vi "DestroyClone.vi"(8 "error in (no error)":errorcluster, 9 "Exit via Stop Module Req?":bool, 10 "Wait for Module to stop?":bool, 11 "ModuleAdmin":refnum<class "ModuleAdmin.lvclass">) -> (0 "error out":errorcluster, 1 "External Launch":bool, 3 "Mod Admin out":refnum<class "ModuleAdmin.lvclass">)   [LabVIEW 2014, in "WfrmModule.lvlib"]
uses:
  WfrmModule.lvlib
  <userlib>/NIST/ModuleAdminLib/ModuleAdmin/ModuleAdmin.lvclass
  <userlib>/NIST/ModuleAdminLib/ModuleAdmin/ModuleAdmin.lvclass/ModuleAdmin.ctl
  <userlib>/NIST/ModuleAdminLib/ModuleAdmin/Accessors/Read CloneRegRef.vi
  <userlib>/NIST/ModuleAdminLib/CloneRegistration/CloneRegistration.lvclass
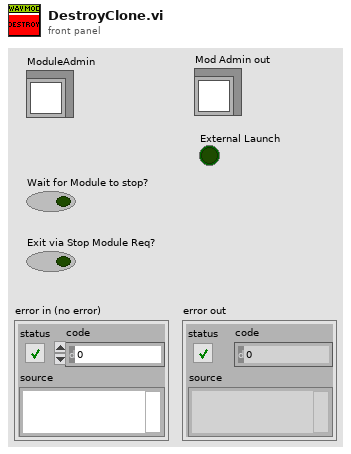
[diagram p1: front panel]
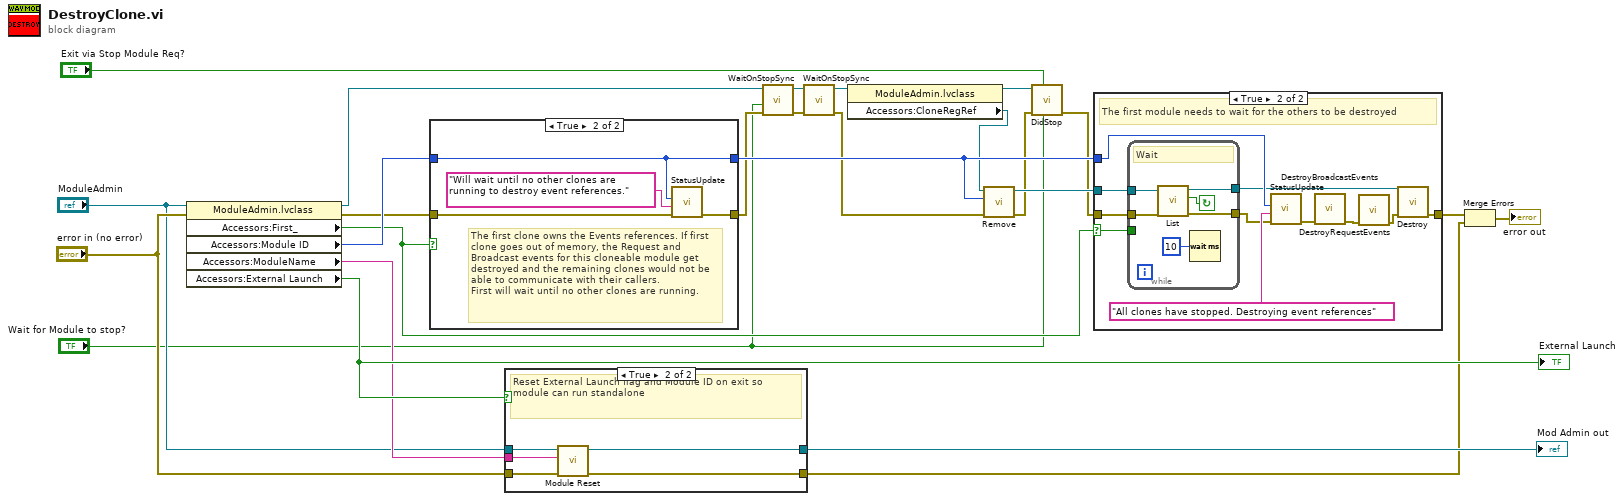
[diagram p0: block diagram]
diagram:
  n1 = property class="ModuleAdmin.lvclass"(reference="ModuleAdmin", error in="error in (no error)") -> (reference out=w4:refnum<class "ModuleAdmin.lvclass">, error out=w7:errorcluster, "Accessors:First_"=w13:bool, "Accessors:Module ID"=w17:i32, "Accessors:ModuleName"=w22:string, "Accessors:External Launch"=w24:bool)
  "External Launch" <- w24
  n2 = case shown="True" w13 {
    tunnel: w7 -> [w27 w31]
    tunnel: w17 -> [w26 w28]
    tunnel: [w27 w29] -> w6
    tunnel: [w26 w28] -> w15
    frame False {
    }
    frame True {
      # "The first clone owns the Events references. If first clone goes out of memory, the Request and Broadcast events for this cloneable module get destroyed and the remaining clones would not be able to communicate with their callers.\nFirst will wait until no other clones are running."
      n3 = call "StatusUpdate.vi"("error in (no error)"=w31, "Status"="Will wait until no other clones are running to destroy event references." ("format string"), "ModuleID"=w28) -> ("error out"=w29:errorcluster)  [unwired: 8 in]
    }
  }
  n4 = case shown="True" w24 {
    tunnel: "error in (no error)" -> [w32 w38]
    tunnel: w22 -> [_ w37]
    tunnel: "ModuleAdmin" -> [w33 w36]
    tunnel: [w33 w35] -> w20
    tunnel: [w32 w34] -> w18
    frame False {
    }
    frame True {
      # "Reset External Launch flag and Module ID on exit so module can run standalone"
      n5 = call <userlib>:"Module Reset.vi"("error in (no error)"=w38, "ModuleName"=w37, "Mod Admin in"=w36) -> ("error out"=w34:errorcluster, "Mod Admin out"=w35:refnum<class "ModuleAdmin.lvclass">)  [unwired: 7 in]
    }
  }
  "Mod Admin out" <- w20
  n6 = call <userlib>:"WaitOnStopSync.vi"("error in (no error)"=w6, "WaitForModuleToStop?"="Wait for Module to stop?", "ModuleAdmin"=w4) -> ("error out"=w25:errorcluster, "ModuleAdmin"=w14:refnum<class "ModuleAdmin.lvclass">)  [unwired: 7 in]
  n7 = call <userlib>:"WaitOnStopSync.vi"("error in (no error)"=w25, "ModuleAdmin"=w14) -> ("error out"=w5:errorcluster, "ModuleAdmin"=w3:refnum<class "ModuleAdmin.lvclass">)  [unwired: 8 in]
  n8 = property class="ModuleAdmin.lvclass"(reference=w3) -> (reference out=w9:refnum<class "ModuleAdmin.lvclass">, "Accessors:CloneRegRef"=w8:refnum<data-value>)  [unwired: 1 in, 1 out]
  n9 = call <userlib>:"Remove.vi"("error in (no error)"=w5, "Module ID"=w15, "CloneRegRef"=w8) -> ("error out"=w11:errorcluster, "CloneRegRef"=w16:refnum<data-value>)  [unwired: 6 in, 1 out]
  n10 = call "DidStop.vi"("Wait for Module to stop?"="Wait for Module to stop?", "Exit via Stop Module Req?"="Exit via Stop Module Req?", "error in (no error)"=w11, "ModuleAdmin"=w9) -> ("error out"=w1:errorcluster)  [unwired: 7 in]
  n11 = case shown="True" w13 {
    selector: w13 -> [_ w50]
    tunnel: w1 -> [w39 w40]
    tunnel: w15 -> [_ w45]
    tunnel: [w39 w43] -> w12
    tunnel: w16 -> [_ w44]
    frame False {
    }
    frame True {
      # "The first module needs to wait for the others to be destroyed"
      n12 = while {
        tunnel: w40 -> [w56]
        tunnel: w50 -> [_]
        tunnel: [w55] -> w48
        tunnel: w44 -> [w52]
        tunnel: [w51] -> w41
        stop <- w54 continue-if-true
        # "Wait"
        n13 = call <userlib>:"List.vi"("error in (no error)"=w56, "CloneRegRef"=w52) -> ("error out"=w55:errorcluster, "Found?"=w54:bool, "CloneRegRef"=w51:refnum<data-value>)  [unwired: 4 in, 3 out]
        n14 = Wait (ms)(milliseconds to wait=u32 10) -> ()  [unwired: 1 out]
      }
      n15 = call "StatusUpdate.vi"("error in (no error)"=w48, "Status"="All clones have stopped. Destroying event references", "ModuleID"=w45) -> ("error out"=w47:errorcluster)  [unwired: 8 in]
      n16 = call "DestroyBroadcastEvents.vi"("error in (no error)"=w47) -> ("error out"=w46:errorcluster)  [unwired: 10 in]
      n17 = call "DestroyRequestEvents.vi"("error in (no error)"=w46) -> ("error out"=w42:errorcluster)  [unwired: 10 in]
      n18 = call <userlib>:"Destroy.vi"("error in (no error)"=w42, "CloneRegRef"=w41) -> ("error out"=w43:errorcluster)  [unwired: 9 in]
    }
  }
  n19 = Merge Errors(w12, w18) -> (→"error out":errorcluster)
